vi "ingest_parquet.vi"(4 "optional":T1, 7 "Timestamp Metadata":refnum<class "timestampMetadata.lvclass">, 8 "error in":errorcluster, 9 "Target":refnum<class "target.lvclass">, 10 "Source":refnum<class "source.lvclass">, 11 "Nominal Client in":refnum<class "Nominal Client.lvclass">) -> (0 "error out":errorcluster, 1 "datasetRid":string, 2 "datasetFileId":string, 3 "Nominal Client out":refnum<class "Nominal Client.lvclass">)   [LabVIEW 2020, in "Nominal Client.lvclass"]
doc: "Triggers an ingest job, allowing either creating a new dataset or uploading to an existing one. This endpoint is meant to supersede all other ingestion endpoints as their functionality gets migrated to this one."
uses:
  Nominal Client.lvclass
  datasources/target/target.lvclass
  datasources/source/source.lvclass
  timestampMetadata/timestampMetadata.lvclass
  Nominal Client.lvclass/Nominal Client.ctl
  datasources/target/target.lvclass/target.ctl
  4e81ab5e-e540-474e-8302-0a664eb7b944.vi
  5b5e685d-1dc7-44a1-a266-f8fb5c0c2742.vi
  eb167d14-4f2b-41c0-88bb-5beef1829223.vi
  datasources/target/workspace.set.vi
  <vilib>/JDP Science/JSONtext/Variant to JSON Text.vi
  <vilib>/JDP Science/JSONtext/support/Format JSON Object.vi
  <vilib>/JDP Science/JSONtext/JSON text to Variant.vi
  <vilib>/JDP Science/JSONtext/LVClass Serializer/JSONtext LVClass Serializer.lvclass
  nominal types/properties/properties.lvclass
  nominal types/labels/labels.lvclass
  <vilib>/JDP Science/JSONtext/JSONtext.lvlib
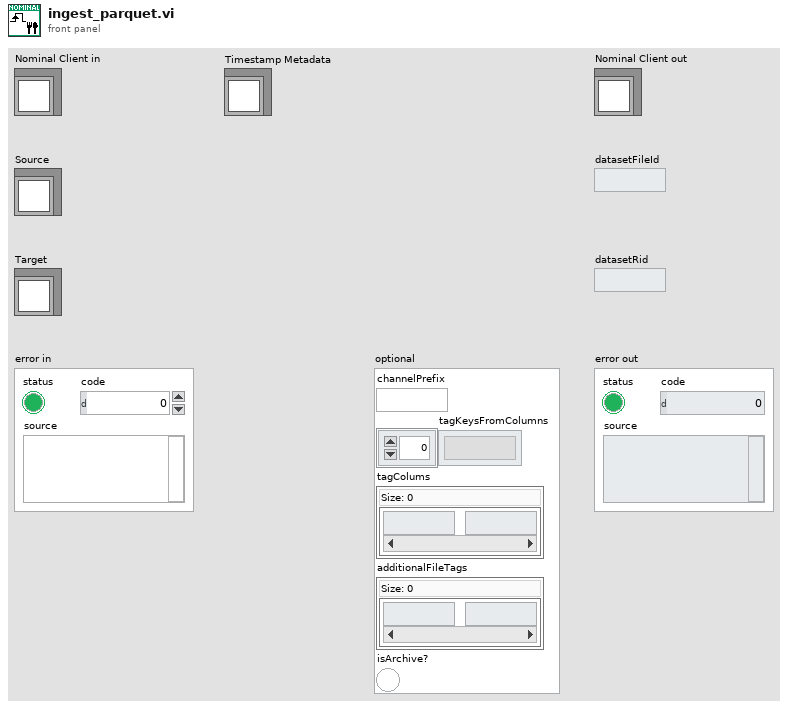
[diagram p1: front panel]
types:
  T1 = cluster{"channelPrefix":string, "tagKeysFromColumns":string[], "tagColums":map{string, string}, "additionalFileTags":map{string, string}, "isArchive?":bool}
  T2 = cluster{"type":string, "dataset":cluster{"datasetFileId":string, "datasetRid":string}}
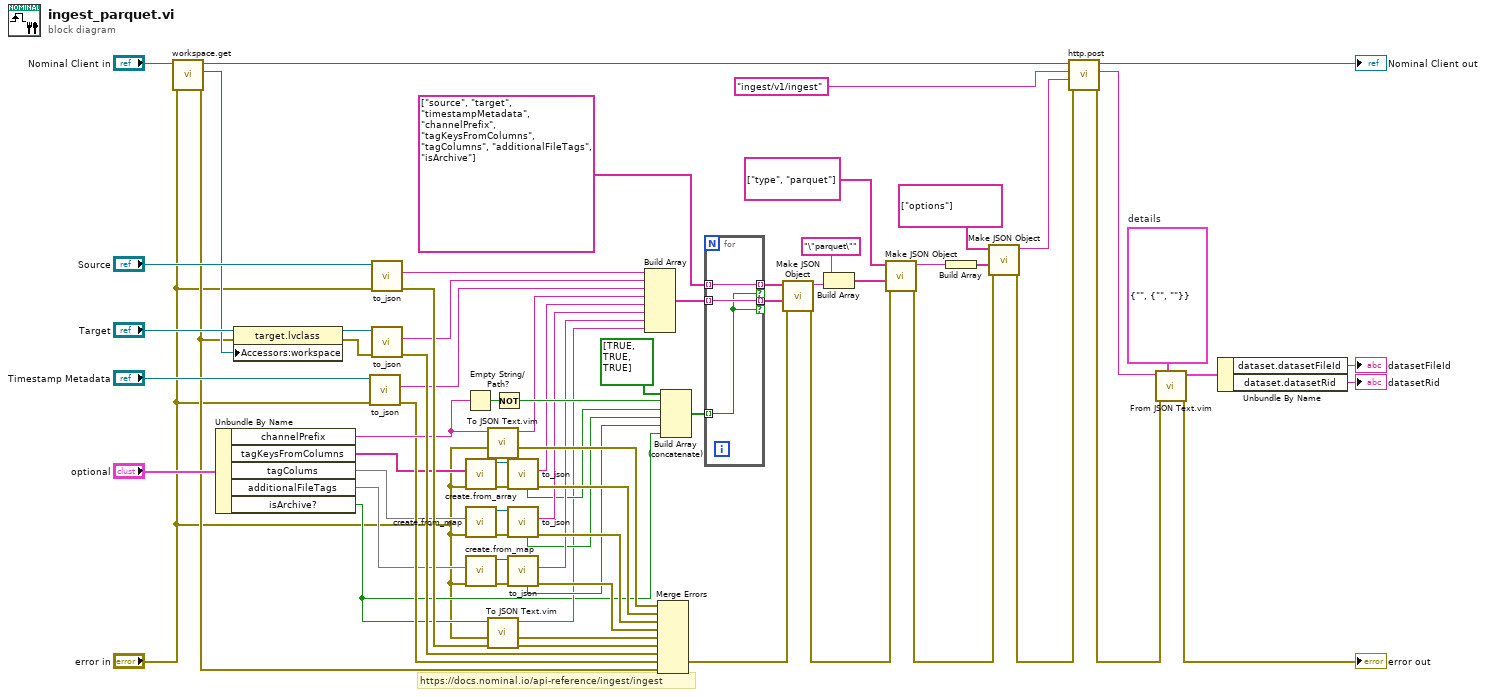
[diagram p0: block diagram]
diagram:
  w23 = T2 {"type"="", "dataset"={"datasetFileId"="", "datasetRid"=""}}  # details
  # "https://docs.nominal.io/api-reference/ingest/ingest"
  n1 = call "workspace.get.vi"("error in"="error in", "Nominal Client in"="Nominal Client in") -> ("error out"=w44:errorcluster, "workspace"=w60:refnum<class "workspace.lvclass">, "Nominal Client out"=w63:refnum<class "Nominal Client.lvclass">)  [unwired: 7 in]
  n2 = Unbundle By Name("optional") -> ("channelPrefix"=w53:string, "tagKeysFromColumns"=w4:string[], "tagColums"=w5:map{string, string}, "additionalFileTags"=w6:map{string, string}, "isArchive?"=w29:bool)
  n3 = property class="target.lvclass"(reference="Target", error in=w44, "Accessors:workspace"=w60) -> (reference out=w65:refnum<class "target.lvclass">, error out=w66:errorcluster)
  n4 = call-dynamic "to_json.vi"("error in"="error in", "timestampMetadata in"="Timestamp Metadata") -> ("error out"=w43:errorcluster, "json"=w56:string)  [unwired: 6 in, 2 out]
  n5 = call-dynamic "to_json.vi"("error in"="error in", "source in"="Source") -> ("error out"=w68:errorcluster, "json"=w58:string)  [unwired: 6 in, 2 out]
  n6 = call-dynamic "to_json.vi"("error in"=w66, "target in"=w65) -> ("error out"=w67:errorcluster, "json"=w57:string)  [unwired: 6 in, 2 out]
  n7 = Empty String/Path?(string/path=w53) -> (empty?=w54:bool)
  n8 = call "create.from_array.vi"("error in"="error in", "labels"=w4) -> ("error out"=w2:errorcluster, "labels out"=w3:refnum<class "labels.lvclass">)  [unwired: 8 in]
  n9 = call "create.from_map.vi"("error in"="error in", "properties"=w5) -> ("error out"=w9:errorcluster, "properties out"=w10:refnum<class "properties.lvclass">)  [unwired: 8 in]
  n10 = call "create.from_map.vi"("error in"="error in", "properties"=w6) -> ("error out"=w7:errorcluster, "properties out"=w8:refnum<class "properties.lvclass">)  [unwired: 8 in]
  n11 = call "To JSON Text.vim"("error in (no error)"="error in", "Anything"=w53) -> ("error out"=w39:errorcluster, "<JSON>"=w38:string)  [unwired: 8 in]
  n12 = call "To JSON Text.vim"("error in (no error)"="error in", "Anything"=w29) -> ("error out"=w31:errorcluster, "<JSON>"=w30:string)  [unwired: 8 in]
  n13 = Not(x=w54) -> (.not. x?=w52:bool)
  n14 = call-dynamic "to_json.vi"("error in"=w2, "labels in"=w3) -> ("error out"=w40:errorcluster, "json"=w37:string, "Not Default"=w34:bool)  [unwired: 6 in, 1 out]
  n15 = call-dynamic "to_json.vi"("error in"=w9, "properties in"=w10) -> ("error out"=w41:errorcluster, "json"=w36:string, "Not Default"=w33:bool)  [unwired: 6 in, 1 out]
  n16 = call-dynamic "to_json.vi"("error in"=w7, "properties in"=w8) -> ("error out"=w42:errorcluster, "json"=w35:string, "Not Default"=w32:bool)  [unwired: 6 in, 1 out]
  n17 = Build Array(w58, w57, w56, w38, w37, w36, w35, w30) -> (w50:string[])
  n18 = Merge Errors(w39, w40, w41, w42, w31, w68, w67, w43, w44) -> (w45:errorcluster)
  n19 = Build Array (concatenate)(bool[] [TRUE, TRUE, TRUE] ("element"), w52, w34, w33, w32, w29) -> (w46:bool[])
  n20 = for {
    tunnel: w50 -> [w73] mode=indexing
    tunnel: [w73] -> w49 mode=indexing if=w71
    tunnel: string[] ["source", "target", "timestampMetadata", "channelPrefix", "tagKeysFromColumns", "tagColumns", "additionalFileTags", "isArchive"] ("Item Names") -> [w72] mode=indexing
    tunnel: [w72] -> w47 mode=indexing if=w71
    tunnel: w46 -> [w71] mode=indexing
  }
  n21 = call <vilib>:"Make JSON Object.vi"("error in (no error)"=w45, "JSON Items"=w49, "Item Names"=w47) -> ("error out"=w24:errorcluster, "<JSON>"=w28:string)  [unwired: 7 in]
  n22 = Build Array("\"parquet\"" ("JSON"), w28) -> (w25:string[])
  n23 = call <vilib>:"Make JSON Object.vi"("error in (no error)"=w24, "JSON Items"=w25, "Item Names"=string[] ["type", "parquet"] ("JSON")) -> ("error out"=w12:errorcluster, "<JSON>"=w14:string)  [unwired: 7 in]
  n24 = Build Array(w14) -> (w16:string[])
  n25 = call <vilib>:"Make JSON Object.vi"("error in (no error)"=w12, "JSON Items"=w16, "Item Names"=string[] ["options"] ("JSON")) -> ("error out"=w11:errorcluster, "<JSON>"=w13:string)  [unwired: 7 in]
  n26 = call "http.post.vi"("error in"=w11, "Request body"=w13, "Path"="ingest/v1/ingest", "Nominal Client in"=w63) -> ("error out"=w18:errorcluster, "Response"=w19:string, "Nominal Client out"=→"Nominal Client out":refnum<class "Nominal Client.lvclass">)  [unwired: 4 in, 1 out]
  n27 = call "From JSON Text.vim"("Data Type and Default Value"=w23, "error in (no error)"=w18, "JSON"=w19) -> ("error out"=→"error out":errorcluster, "Data out"=w22:T2)  [unwired: 7 in]
  n28 = Unbundle By Name(w22) -> ("dataset.datasetFileId"=→"datasetFileId":string, "dataset.datasetRid"=→"datasetRid":string)
